vi "test_tcp.vi"() -> ()   [LabVIEW 2014]
panel:
  out "IP":string
  out "错误输出":errorcluster
  out "数据输出":string
  in  "停止":bool
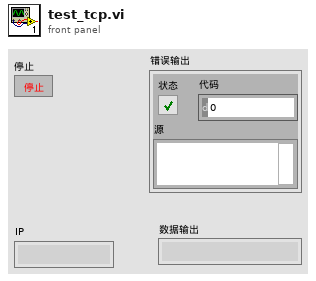
[diagram p1: front panel]
types:
  T1 = enum16{"Standard", "Buffered", "CRLF", "Immediate"}
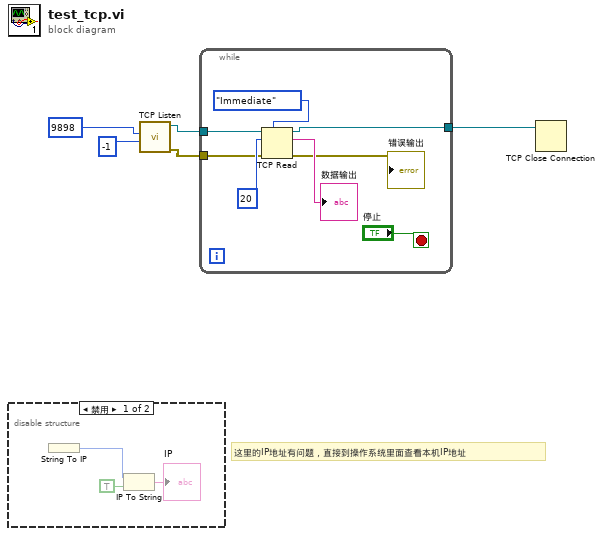
[diagram p0: block diagram]
diagram:
  # "这里的IP地址有问题，直接到操作系统里面查看本机IP地址"
  n1 = disable-structure shown="禁用" {
    frame Disabled {
      n2 = String To IP() -> (0:w8:u32)  [unwired: 1 in]
      n3 = IP To String(1:TRUE ("句点符号？(F)"), 2:w8) -> (0:→"IP":string)
    }
    frame Enabled {
    }
  }
  n4 = call <vilib>:"TCP Listen.vi"("timeout ms (wait forever: -1)"=-1, "port"=u16 9898) -> ("error out"=w1:errorcluster, "connection ID"=w5:refnum<k5>)  [unwired: 5 in, 3 out]
  n5 = while {
    tunnel: w5 -> [w16]
    tunnel: [w15] -> w4
    tunnel: w1 -> [w10]
    stop <- "停止" stop-if-true
    n6 = TCP Read(connection ID=w16, bytes to read=20 ("读取的字节"), error in (no error)=w10, 7:T1."Immediate" ("模式（标准）")) -> (connection ID out=w15:refnum<k5>, data out=→"数据输出":string, error out=→"错误输出":errorcluster)  [unwired: 1 in]
  }
  n7 = TCP Close Connection(connection ID=w4) -> ()  [unwired: 2 in, 2 out]
